vi "BT Example 5 - Selector.vi"() -> ()   [LabVIEW 2021]
uses:
  Support/Nodes/abs_Node/Status.ctl
  Blackboard/Blackboard.lvclass
  Support/Nodes/Decorators/Repeater/Support/Finish On - Type.ctl
  System/bt_System.lvclass
  Blackboard/Blackboard.lvclass/Blackboard.ctl
  Support/Nodes/Leaves/abs_Type Leaf/abs_Type Leaf.lvclass/abs_Type Leaf.ctl
  Blackboard/Get Value Type/Get I32.vi
  <vilib>/TSA/Abstract Data Classes/Abs_Types/I32 Integer/Static Read.vi
  Blackboard/Support/Index Group.vi
  Blackboard/Support/Index Tags.vi
  Support/Nodes/Leaves/abs_Type Leaf/Properties/Write Value Class.vi
  <vilib>/TSA/Omni-Bus/Local Bus/Support/I32/Local Bus_I32.lvclass
  C:/Program Files (x86)/National Instruments/LabVIEW 2021/vi.lib/TSA/Abstract Data Classes/Abs_Types/Value/Abs_Value.lvclass
  <vilib>/TSA/Abstract Data Classes/Abs_Types/I32 Integer/Abs_I32 Integer.lvclass
  Support/Nodes/Leaves/Test Boolean/Test Abs_Boolean.lvclass
  C:/Users/Tim/Documents/GitHub/LV_Behaviour_Tree/Source/Support/Nodes/abs_Node/bt_Node.lvclass
  C:/Users/Tim/Documents/GitHub/LV_Behaviour_Tree/Source/Support/Nodes/Leaves/abs_Type Leaf/abs_Type Leaf.lvclass
  <vilib>/TSA/Abstract Data Classes/Abs_Types/Boolean/Abs_Boolean.lvclass
  C:/Program Files (x86)/National Instruments/LabVIEW 2021/vi.lib/TSA/Abstract Data Classes/Abs_Types/Type/Abs_Type.lvclass
  <vilib>/TSA/Omni-Bus/Local Bus/Support/Initialise DVR's.vi
  <vilib>/TSA/Abstract Data Classes/Functions/Math/Support/Increment/I32/Method.vi
  <vilib>/TSA/Abstract Data Classes/Abs_Types/Value/Abs_Value.lvclass
  <vilib>/TSA/Abstract Data Classes/Abs_Types/Type/Abs_Type.lvclass
  <vilib>/TSA/Omni-Bus/Local Bus/Support/DBL/Local Bus_DBL.lvclass
  <vilib>/TSA/Omni-Bus/Local Bus/Support/SGL/Local Bus_SGL.lvclass
  <vilib>/TSA/Omni-Bus/Local Bus/Support/EXT/Local Bus_EXT.lvclass
  <vilib>/TSA/Omni-Bus/Local Bus/Support/Bool/Local Bus_Boolean.lvclass
  <vilib>/TSA/Omni-Bus/Local Bus/Support/STR/Local Bus_String.lvclass
  <vilib>/TSA/Omni-Bus/Local Bus/Support/Variant/Local Bus_Variant.lvclass
  <vilib>/TSA/Omni-Bus/Local Bus/Support/WFM/Local Bus_Waveform.lvclass
  <vilib>/TSA/Omni-Bus/Local Bus/Support/Time/Local Bus_Time.lvclass
  <vilib>/TSA/Omni-Bus/Local Bus/Support/U8/Local Bus_U8.lvclass
  <vilib>/TSA/Omni-Bus/Local Bus/Support/U16/Local Bus_U16.lvclass
  <vilib>/TSA/Omni-Bus/Local Bus/Support/U32/Local Bus_U32.lvclass
  <vilib>/TSA/Omni-Bus/Local Bus/Support/U64/Local Bus_U64.lvclass
  <vilib>/TSA/Omni-Bus/Local Bus/Support/I8/Local Bus_I8.lvclass
  <vilib>/TSA/Omni-Bus/Local Bus/Support/I16/Local Bus_I16.lvclass
  <vilib>/TSA/Omni-Bus/Local Bus/Support/I64/Local Bus_I64.lvclass
  <vilib>/TSA/Omni-Bus/Local Bus/Support/CSGL/Local Bus_CSGL.lvclass
  <vilib>/TSA/Omni-Bus/Local Bus/Support/CDBL/Local Bus_CDBL.lvclass
  <vilib>/TSA/Omni-Bus/Local Bus/Support/CEXT/Local Bus_CEXT.lvclass
  <vilib>/TSA/Abstract Data Classes/Functions/Compare/Support/Less/I32/Method_Const.vi
  <vilib>/TSA/Abstract Data Classes/Constants/Support/I32/I32.vi
  BT.lvlib
  Support/Nodes/Decorators/Repeater/bt_Repeater.lvclass
  Support/Nodes/abs_Node/bt_Node.lvclass
  <vilib>/TSA/Abstract Data Classes/Functions/Math/Support/Increment/I32/Increment_I32.lvclass
  <vilib>/TSA/Abstract Data Classes/Functions/Compare/Support/Less/I32/Less_I32.lvclass
  <vilib>/TSA/Abstract Data Classes/Constants/Support/I32/Const_I32.lvclass
panel:
  out "Failure Count":i32
  out "Count":i32
  out "Status":T1
  in  "stop":bool
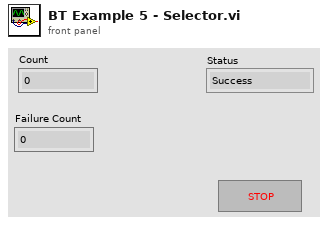
[diagram p1: front panel]
types:
  T1 = typedef "BT.lvlib/bt_Node.lvclass/Status.ctl" = enum16{"Success", "Failure", "Running"}
  T2 = typedef "BT.lvlib/bt_Repeater.lvclass/Finish On - Type.ctl" = enum16{"Success", "Failure", "Never"}
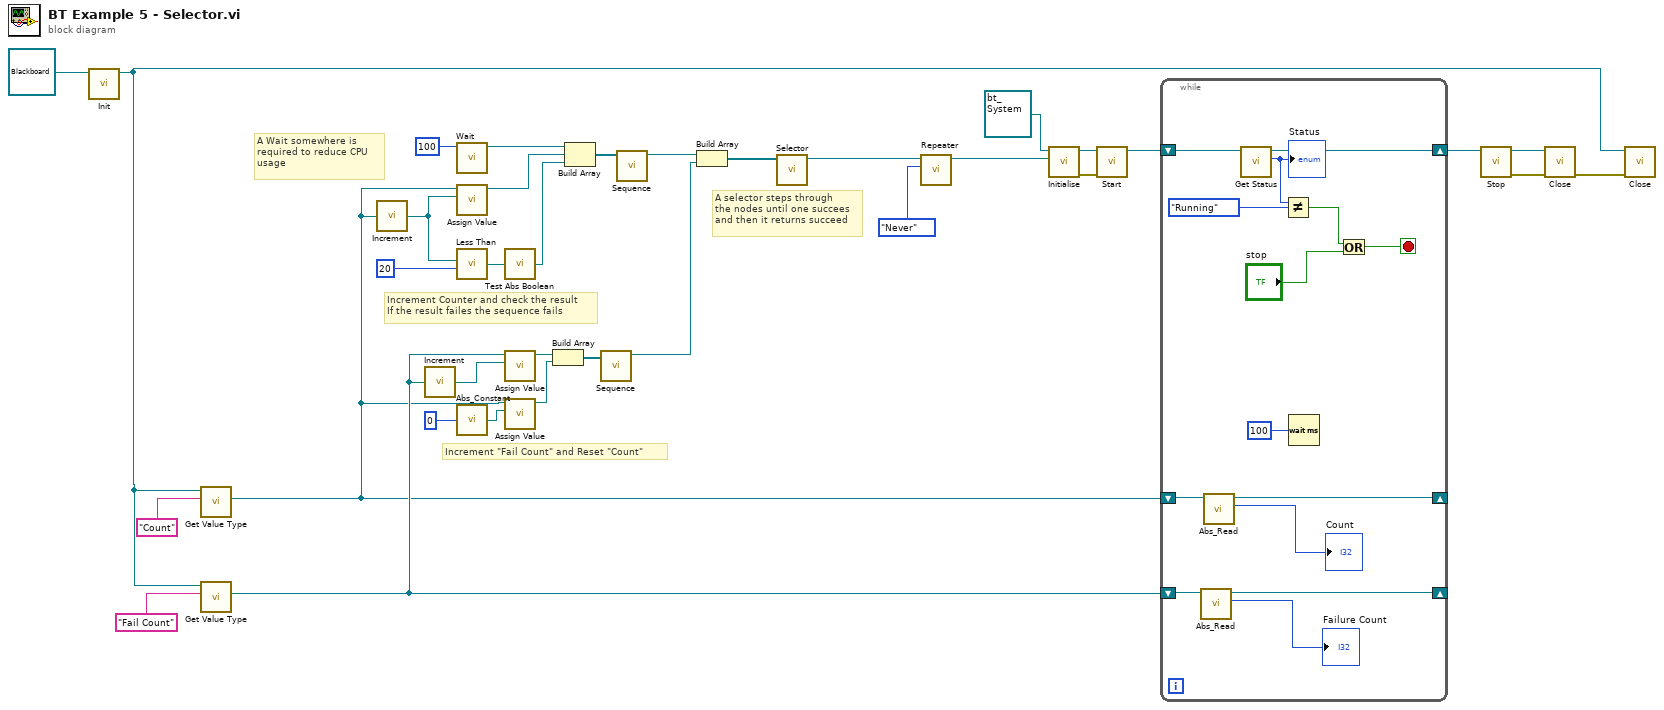
[diagram p0: block diagram]
diagram:
  # "A Wait somewhere is\nrequired to reduce CPU \nusage"
  # "Increment \"Fail Count\" and Reset \"Count\""
  # "A selector steps through\nthe nodes until one succees\nand then it returns succeed"
  # "Increment Counter and check the result\nIf the result failes the sequence fails"
  n1 = call-dynamic "Init.vi"("bt_Blackboard in"=refnum<class "Blackboard.lvclass"> refnum) -> ("bt_Blackboard out"=w12:refnum<class "Blackboard.lvclass">)  [unwired: 9 in, 1 out]
  n2 = call-poly "Get Value Type.vi"("Tag"="Count", "Blackboard in"=w12) -> ("Value"=w3:refnum<class "Abs_I32 Integer.lvclass">)  [unwired: 6 in, 3 out]
  n3 = call-poly "Get Value Type.vi"("Tag"="Fail Count", "Blackboard in"=w12) -> ("Value"=w10:refnum<class "Abs_I32 Integer.lvclass">)  [unwired: 6 in, 3 out]
  n4 = call-poly <vilib>:"Increment.vi"("Value"=w3) -> ("Result"=w19:refnum<class "Abs_I32 Integer.lvclass">)  [unwired: 4 in]
  n5 = call-poly <vilib>:"Increment.vi"("Value"=w10) -> ("Result"=w11:refnum<class "Abs_I32 Integer.lvclass">)  [unwired: 4 in]
  n6 = call "Wait.vi"("Time (ms)"=u32 100) -> ("Node Out"=w9:refnum<class "bt_Node.lvclass">)  [unwired: 10 in]
  n7 = call "Assign Value.vi"("Assigned Value"=w19, "Value"=w3) -> ("Node Out"=w16:refnum<class "bt_Node.lvclass">)  [unwired: 9 in]
  n8 = call-poly <vilib>:"Less Than.vi"("Value"=20, "Value A"=w19) -> ("Result"=w20:refnum<class "Abs_Boolean.lvclass">)  [unwired: 4 in]
  n9 = call-poly <vilib>:"Abs_Constant.vi"("Value"=0) -> ("Constant"=w2:refnum<class "Abs_I32 Integer.lvclass">)  [unwired: 4 in]
  n10 = call "Test Abs Boolean.vi"("Abs_Boolean.lvclass"=w20) -> ("abs_Node"=w15:refnum<class "bt_Node.lvclass">)  [unwired: 4 in]
  n11 = call "Assign Value.vi"("Assigned Value"=w11, "Value"=w10) -> ("Node Out"=w7:refnum<class "bt_Node.lvclass">)  [unwired: 9 in]
  n12 = call "Assign Value.vi"("Assigned Value"=w2, "Value"=w3) -> ("Node Out"=w4:refnum<class "bt_Node.lvclass">)  [unwired: 9 in]
  n13 = Build Array(w7, w4) -> (w6:refnum<class "bt_Node.lvclass">[])
  n14 = Build Array(w9, w16, w15) -> (w17:refnum<class "bt_Node.lvclass">[])
  n15 = call "Sequence.vi"("Nodes"=w6) -> ("Node"=w5:refnum<class "bt_Node.lvclass">)  [unwired: 10 in]
  n16 = call "Sequence.vi"("Nodes"=w17) -> ("Node"=w14:refnum<class "bt_Node.lvclass">)  [unwired: 10 in]
  n17 = Build Array(w14, w5) -> (w22:refnum<class "bt_Node.lvclass">[])
  n18 = call "Selector.vi"("Nodes"=w22) -> ("Node"=w23:refnum<class "bt_Node.lvclass">)  [unwired: 10 in]
  n19 = call "Repeater.vi"("Finish On"=Finish_On_-_Type."Never", "Node In"=w23) -> ("Node Out"=w25:refnum<class "bt_Node.lvclass">)  [unwired: 9 in]
  n20 = call "Initialise.vi"("Behaviour Tree"=w25, "bt_System in"=refnum<class "bt_System.lvclass"> refnum) -> ("error out"=w26:errorcluster, "bt_System out"=w27:refnum<class "bt_System.lvclass">)  [unwired: 8 in]
  n21 = call "Start.vi"("error in (no error)"=w26, "bt_System in"=w27) -> ("bt_System out"=w34:refnum<class "bt_System.lvclass">)  [unwired: 8 in, 1 out]
  n22 = while {
    shift-right: [w46] -> w33
    shift-left: w34 -> [w47]
    shift-right: [w38] -> _
    shift-left: w3 -> [w39]
    shift-right: [w37] -> _
    shift-left: w10 -> [w36]
    stop <- w44 stop-if-true
    n23 = call-poly <vilib>:"Abs_Read.vi"("Abs_I32 Integer in"=w36) -> ("Value"=→"Failure Count":i32, "Abs_I32 Integer out"=w37:refnum<class "Abs_I32 Integer.lvclass">)  [unwired: 8 in, 1 out]
    n24 = call-poly <vilib>:"Abs_Read.vi"("Abs_I32 Integer in"=w39) -> ("Value"=→"Count":i32, "Abs_I32 Integer out"=w38:refnum<class "Abs_I32 Integer.lvclass">)  [unwired: 8 in, 1 out]
    n25 = call "Get Status.vi"("bt_System in"=w47) -> ("Status"=w43:T1, "bt_System out"=w46:refnum<class "bt_System.lvclass">)  [unwired: 8 in, 1 out]
    "Status" <- w43
    n26 = Not Equal?(x=w43, y=Status."Running") -> (x != y?=w41:bool)
    n27 = Wait (ms)(milliseconds to wait=u32 100) -> ()  [unwired: 1 out]
    n28 = Or(x=w41, y="stop") -> (x .or. y?=w44:bool)
  }
  n29 = call "Stop.vi"("bt_System in"=w33) -> ("error out"=w28:errorcluster, "bt_System out"=w29:refnum<class "bt_System.lvclass">)  [unwired: 9 in]
  n30 = call-dynamic "Close.vi"("error in (no error)"=w28, "bt_System in"=w29) -> ("error out"=w32:errorcluster)  [unwired: 8 in, 1 out]
  n31 = call-dynamic "Close.vi"("error in (no error)"=w32, "bt_Blackboard in"=w12) -> ()  [unwired: 8 in, 2 out]
